vi "data_getWaveSubset.vi"(8 "error in (no error)":errorcluster, 9 "length":u64, 10 "index":u64, 11 "Waveform":waveform(dbl)) -> (0 "error out":errorcluster, 3 "Waveform out":waveform(dbl))   [LabVIEW 2020, in "NI_ExcelFile.lvlib"]
uses:
  <vilib>/express/express shared/NI_ExcelFile/NI_ExcelFile.lvlib
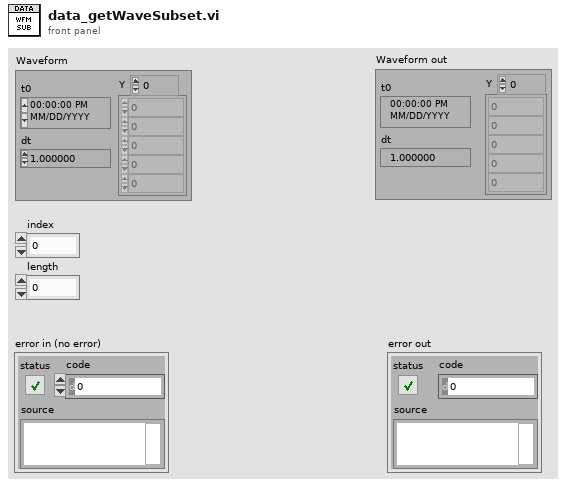
[diagram p1: front panel]
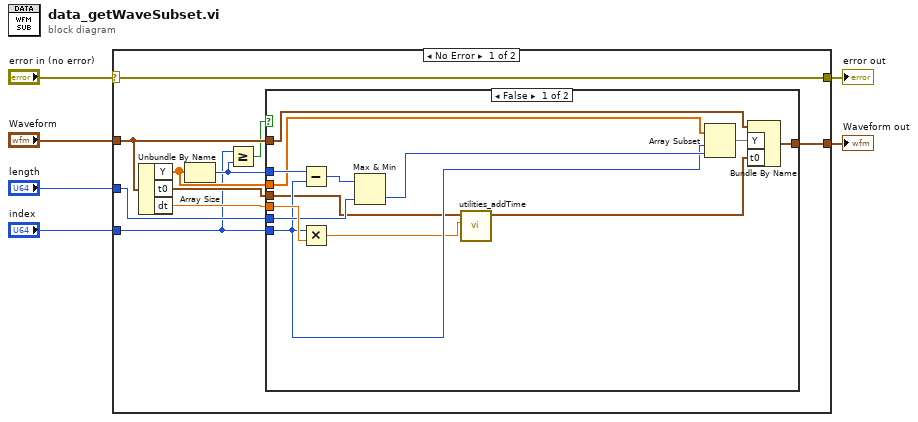
[diagram p0: block diagram]
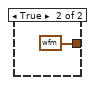
[diagram p2: hidden frame]
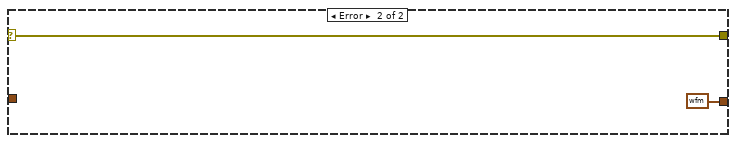
[diagram p3: hidden frame]
diagram:
  n1 = case shown="No Error" "error in (no error)" {
    selector: "error in (no error)" -> [w9 w32]
    tunnel: "index" -> [w8 _]
    tunnel: "length" -> [w16 _]
    tunnel: [w14 waveform(dbl) {"t0"=timestamp(0 s since 1904-01-01), "dt"=1.0, "Y"=[]} ("waveform out")] -> w4
    tunnel: "Waveform" -> [w12 _]
    tunnel: [w9 w32] -> w1
    frame No Error {
      n2 = Unbundle By Name(w12) -> ("Y"=w13:dbl[], "t0"=w11:timestamp, "dt"=w10:dbl)
      n3 = Array Size(array=w13) -> (size(s)=w15:i32)
      n4 = Greater Or Equal?(x=w8, y=w15) -> (x >= y?=w7:bool)
      n5 = case shown="False" w7 {
        tunnel: [w23 waveform(dbl) {"t0"=timestamp(0 s since 1904-01-01), "dt"=1.0, "Y"=[]} ("waveform out")] -> w14
        tunnel: w16 -> [w21 _]
        tunnel: w15 -> [w29 _]
        tunnel: w8 -> [w20 _]
        tunnel: w13 -> [w28 _]
        tunnel: w12 -> [w26 _]
        tunnel: w11 -> [w19 _]
        tunnel: w10 -> [w24 _]
        frame False {
          n6 = Subtract(x=w29, y=w20) -> (x-y=w22:u64)
          n7 = Multiply(x=w20, y=w24) -> (x*y=w18:dbl)
          n8 = Max & Min(x=w22, y=w21) -> (min(x,y)=w27:u64)  [unwired: 1 out]
          n9 = call <vilib>:"utilities_addTime.vi"("number"=w18, "Time"=w19) -> ("Time out"=w17:timestamp)  [unwired: 9 in]
          n10 = Array Subset(array=w28, index=w20, length=w27) -> (w25:dbl[])
          n11 = Bundle By Name(cluster=w26, "Y"=w25, "t0"=w17) -> (w23:waveform(dbl))
        }
        frame True {
        }
      }
    }
    frame Error {
    }
  }
  "Waveform out" <- w4
  "error out" <- w1
